vi "LVIS_Message.vi"(8 "Error In":errorcluster, 11 "Msg State":T1) -> (0 "Error Out":errorcluster)   [LabVIEW 2015]
doc: "Displays a message to the user."
uses:
  Ctrls/LVIS_Msg State.ctl
  Globals/LVIS_DcGlobals.vi
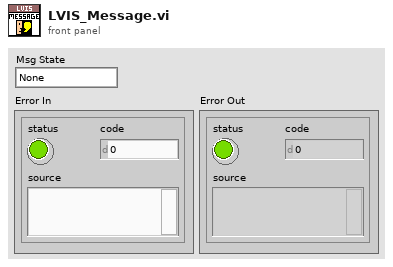
[diagram p1: front panel]
types:
  T1 = typedef "LVIS_Msg State.ctl" = enum16{"None", "Offline", "Online", "Backup Full"}
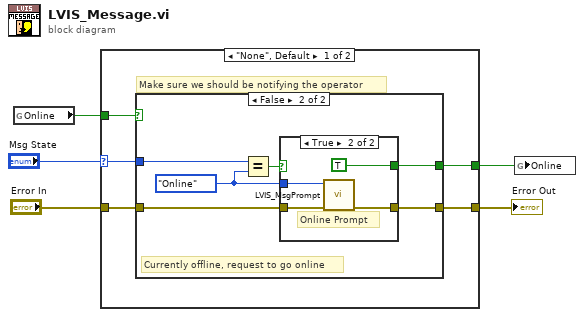
[diagram p0: block diagram]
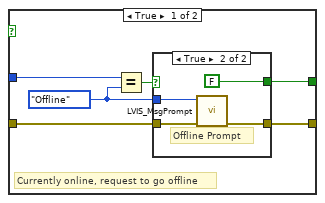
[diagram p2: hidden frame]
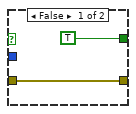
[diagram p3: hidden frame]
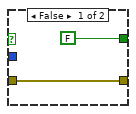
[diagram p4: hidden frame]
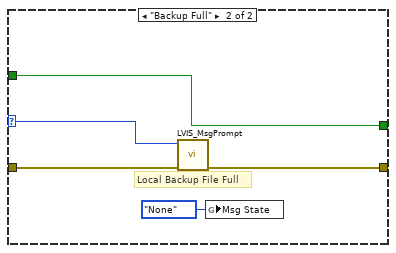
[diagram p5: hidden frame]
diagram:
  n1 = global read "LVIS_DcGlobals.vi" "Online"() -> (w3:bool)
  n2 = case shown="\"None\", Default" "Msg State" {
    selector: "Msg State" -> [w6 w36]
    tunnel: "Error In" -> [w10 w39]
    tunnel: [w9 w38] -> w4
    tunnel: w3 -> [w8 w37]
    tunnel: [w7 w37] -> w2
    frame "None", Default {
      # "Make sure we should be notifying the operator"
      n3 = case shown="False" w8 {
        tunnel: w10 -> [w16 w28]
        tunnel: [w15 w27] -> w9
        tunnel: w6 -> [w14 w26]
        tunnel: [w12 w24] -> w7
        frame True {
          w11 = LVIS_Msg_State."Offline" ("Msg State")
          # "Currently online, request to go offline"
          n4 = Equal?(x=w14, y=w11) -> (x = y?=w13:bool)
          n5 = case shown="True" w13 {
            tunnel: w16 -> [w18 w22]
            tunnel: [w18 w21] -> w15
            tunnel: w11 -> [_ w20]
            tunnel: [TRUE FALSE] -> w12
            frame False {
            }
            frame True {
              # "Offline Prompt"
              n6 = call "LVIS_MsgPrompt.vi"("Error In"=w22, "Msg State"=w20) -> ("Error Out"=w21:errorcluster)  [unwired: 9 in]
            }
          }
        }
        frame False {
          w23 = LVIS_Msg_State."Online" ("Msg State")
          # "Currently offline, request to go online"
          n7 = Equal?(x=w26, y=w23) -> (x = y?=w25:bool)
          n8 = case shown="True" w25 {
            tunnel: w28 -> [w30 w34]
            tunnel: [w30 w33] -> w27
            tunnel: w23 -> [_ w32]
            tunnel: [FALSE TRUE] -> w24
            frame False {
            }
            frame True {
              # "Online Prompt"
              n9 = call "LVIS_MsgPrompt.vi"("Error In"=w34, "Msg State"=w32) -> ("Error Out"=w33:errorcluster)  [unwired: 9 in]
            }
          }
        }
      }
    }
    frame "Backup Full" {
      # "Local Backup File Full"
      n10 = call "LVIS_MsgPrompt.vi"("Error In"=w39, "Msg State"=w36) -> ("Error Out"=w38:errorcluster)  [unwired: 9 in]
      n11 = global write "LVIS_DcGlobals.vi" "Msg State"(LVIS_Msg_State."None" ("Msg State")) -> ()
    }
  }
  "Error Out" <- w4
  n12 = global write "LVIS_DcGlobals.vi" "Online"(w2) -> ()
